vi "Stop Core.vi"(10 "final error code":i32, 11 "Assert in":refnum<class "Assert.lvclass">) -> (3 "Assert out":refnum<class "Assert.lvclass">)   [LabVIEW 2019, in "Assert.lvlib" / "Assert.lvclass"]
doc: "(<B>Filename</B>: Actor Framework.lvlib:Actor.lvclass:Stop Core.vi)\n\nDefines what the actor does before it stops. Use the <B>final error code</B> input to determine whether the actor shut down in response to an error.\n\nBy default, this method passes the Stop message along to all auto-stop nested actors. A descendant class may override this method to define additional behavior, such as shutting down any processes the actor initiated in its override of the Actor Core method."
uses:
  Assert.lvclass
  Assert.lvclass/Assert.ctl
  <vilib>/NI/Event Source Actor/Event Source/Event Source/Event Source.lvclass
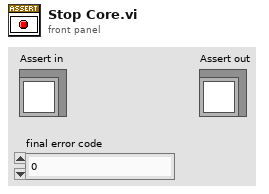
[diagram p1: front panel]
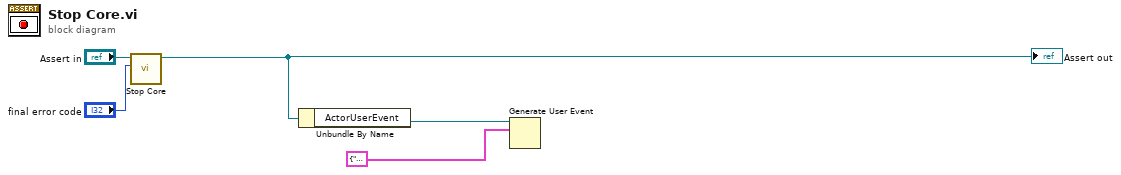
[diagram p0: block diagram]
diagram:
  n1 = call-parent "Stop Core.vi"("final error code"="final error code", "Event Source In"="Assert in") -> ("Event Source Out"=w3:refnum<class "Assert.lvclass">)  [unwired: 9 in]
  "Assert out" <- w3
  n2 = Unbundle By Name(w3) -> ("ActorUserEvent"=w2:refnum<user-event>)
  n3 = Generate User Event(user event=w2, event data cluster=cluster{"Massage":string, "Value":string} {"Massage"="Exit", "Value"=""} ("event data")) -> ()  [unwired: 2 in, 2 out]
